vi "PID_Noise.vi"() -> ()   [LabVIEW 2021]
uses:
  <vilib>/addons/control/pid/pid.llb/PID (DBL).vi
  <vilib>/addons/control/pid/NI_PID_pid.lvlib
panel:
  in  "milliseconds to wait":u32
  out "Waveform Chart":dbl(graph)
  in  "setpoint":dbl format="%.2f"
  in  "stop":bool
  out "process variable":dbl format="%.2f"
  in  "PID gains":T1={"proportional gain (Kc)"=1.0, "integral time (Ti, min)"=0.01, "derivative time (Td, min)"=0.0} {"derivative time (Td, min)" format="%.3f"; "integral time (Ti, min)" format="%.3f"; "proportional gain (Kc)" format="%.3f"}
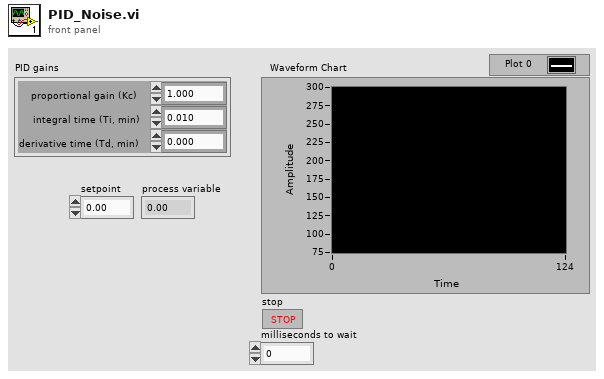
[diagram p1: front panel]
types:
  T1 = cluster{"proportional gain (Kc)":dbl, "integral time (Ti, min)":dbl, "derivative time (Td, min)":dbl}
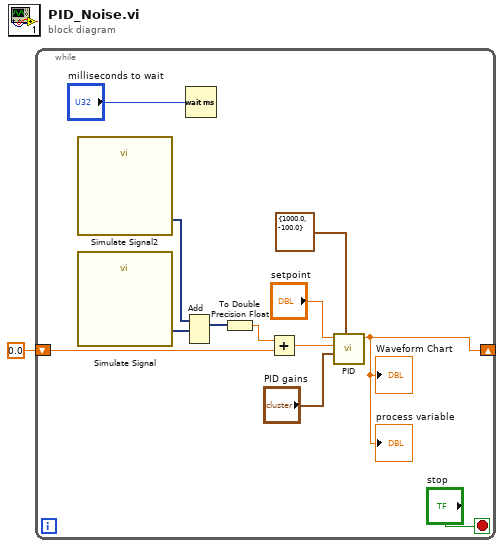
[diagram p0: block diagram]
diagram:
  n1 = while {
    shift-right: [w4] -> _
    shift-left: 0.0 -> [w7]
    stop <- "stop" stop-if-true
    n2 = call "Simulate Signal2"() -> ("DC with Uniform Noise"=w11:dynamicdata)  [unwired: 14 in, 1 out]
    n3 = call "Simulate Signal"() -> ("Sine"=w10:dynamicdata)  [unwired: 14 in, 1 out]
    n4 = Add(1:w10, 2:w11) -> (0:w9:dynamicdata)  [unwired: 1 in, 1 out]
    n5 = Wait (ms)(milliseconds to wait="milliseconds to wait") -> ()  [unwired: 1 out]
    n6 = To Double Precision Float(number=w9) -> (double precision float=w8:dbl)
    n7 = Add(x=w8, y=w7) -> (x+y=w6:dbl)
    n8 = call-poly <vilib>:"PID.vi"("output range"=cluster{"output high":dbl, "output low":dbl} {"output high"=1000.0, "output low"=-100.0}, "PID gains"="PID gains", "process variable"=w6, "setpoint"="setpoint") -> ("output"=w4:dbl)  [unwired: 6 in, 1 out]
    "process variable" <- w4
    "Waveform Chart" <- w4
  }
